vi "Euclidean_distances.vi"(6 "Type Y":T1(ring), 7 "Type X":T1(ring), 8 "error in":errorcluster caption="entrée d'erreur", 9 "Y":string[][](array[string]), 10 "X":string[][](array[string]), 11 "euclidean_distances":T3) -> (0 "error out":errorcluster caption="sortie d'erreur", 3 "Data":T2)   [LabVIEW 2020]
doc: "Considering the rows of X (and Y=X) as vectors, compute the distance matrix between each pair of vectors.\n\nFor efficiency reasons, the euclidean distance between a pair of row vector x and y is computed as :\n\ndist(x, y) = sqrt(dot(x, x) - 2 * dot(x, y) + dot(y, y))\n\nThis formulation has two advantages over other ways of computing distances. First, it is computationally efficient when dealing with sparse data. Second, if one argument varies but the other remains unchanged, then dot(x, x) and/or dot(y, y) can be pre-computed.\n\nHowever, this is not the most precise way of doing this computation, and the distance matrix returned by this function may not be exactly symmetric as required by, e.g., scipy.spatial.distance functions.\n\n\nParameters :\n\n- X : {array-like, sparse matrix}, shape (n_samples_1, n_features)\n\n- Y : {array-like, sparse matrix}, shape (n_samples_2, n_features)\n\n- Y_norm_squared : array-like, shape (n_samples_2, ), optional\nPre-computed dot-products of vectors in Y (e.g., (Y**2).sum(axis=1)) May be ignored in some cases, see the note below.\n\n- squared : boolean, optional\nReturn squared Euclidean distances.\n\n- X_norm_squared : array-like of shape (n_samples,), optional\nPre-computed dot-products of vectors in X (e.g., (X**2).sum(axis=1)) May be ignored in some cases, see the note below.\n\nReturns : \n\n- distances : array, shape (n_samples_1, n_samples_2)"
uses:
  Euclidean_distances.lvclass
panel:
  out "Euclidean_distances.lvclass":refnum<class "Euclidean_distances.lvclass">
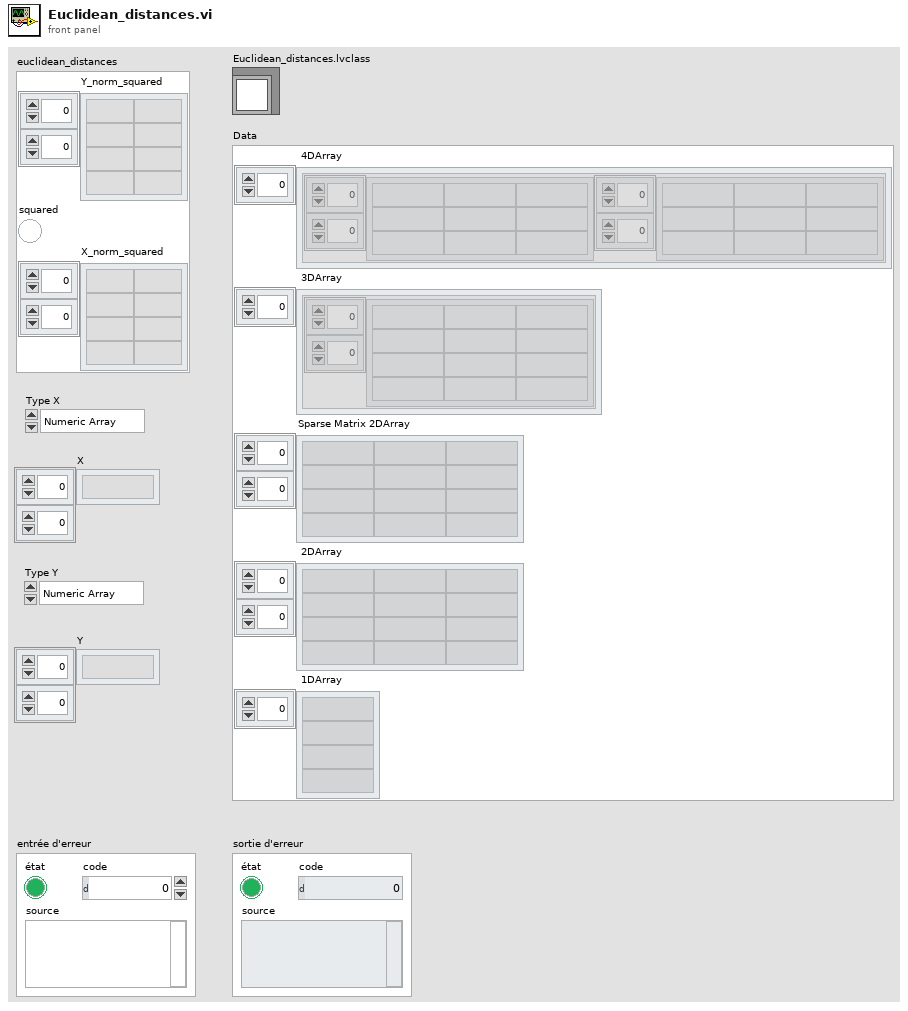
[diagram p1: front panel]
types:
  T1 = enum16{"Numeric Array", "String Array", "Sparse"}
  T2 = cluster{" 4DArray":cluster{"1":string[][], "2":string[][]}[], " 3DArray":cluster{"Tableau":string[][]}[], "Sparse Matrix 2DArray":string[][], " 2DArray":string[][], " 1DArray":string[]}
  T3 = cluster{"Y_norm_squared":string[][], "squared":bool, "X_norm_squared":string[][]}
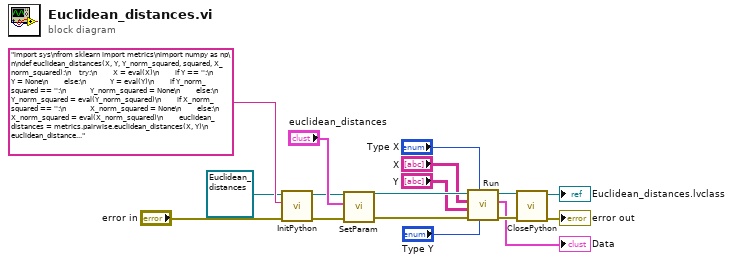
[diagram p0: block diagram]
diagram:
  n1 = call-dynamic "InitPython.vi"("error in (no error)"="error in", "Python Instruction"="import sys\nfrom sklearn import metrics\nimport numpy as np\n\ndef euclidean_distances(X, Y, Y_norm_squared, squared, X_norm_squared):\n    try:\n        X = eval(X)\n        if Y == '':\n            Y = None\n        else:\n            Y = eval(Y)\n        if Y_norm_squared == '':\n            Y_norm_squared = None\n        else:\n            Y_norm_squared = eval(Y_norm_squared)\n        if X_norm_squared == '':\n            X_norm_squared = None\n        else:\n            X_norm_squared = eval(X_norm_squared)\n        euclidean_distances = metrics.pairwise.euclidean_distances(X, Y)\n        euclidean_distances = euclidean_distances.tolist()\n        return str(euclidean_distances)\n    except:\n        erreur = sys.exc_info()\n        typerr = u\"%s\" % (erreur[0])\n        typerr = typerr[typerr.find(\"'\")+1:typerr.rfind(\"'\")]\n        msgerr = u\"%s\" % (erreur[1])\n        message = str('/!\\\\ {0} : {1}'. format(typerr,msgerr))\n        return message", "Scikit-learn en entrée"=refnum<class "Euclidean_distances.lvclass"> refnum ("Euclidean_distances.lvclass")) -> ("error out"=w13:errorcluster, "Scikit-learn en sortie"=w12:refnum<class "Euclidean_distances.lvclass">)  [unwired: 7 in]
  n2 = call-dynamic "SetParam.vi"("error in (no error)"=w13, "euclidean_distances"="euclidean_distances", "Euclidean_distances.lvclass"=w12) -> ("error out"=w8:errorcluster, "Euclidean_distances.lvclass"=w9:refnum<class "Euclidean_distances.lvclass">)  [unwired: 7 in]
  n3 = call-dynamic "Run.vi"("Type Y"="Type Y", "Type X"="Type X", "error in (no error)"=w8, "Y"="Y", "X"="X", "Euclidean_distances.lvclass"=w9) -> ("error out"=w10:errorcluster, "Data"=→"Data":T2, "Euclidean_distances.lvclass"=w11:refnum<class "Euclidean_distances.lvclass">)  [unwired: 3 in]
  n4 = call-dynamic "ClosePython.vi"("error in (no error)"=w10, "Scikit-learn en entrée"=w11) -> ("error out"=→"error out":errorcluster, "Scikit-learn en sortie"=→"Euclidean_distances.lvclass":refnum<class "Euclidean_distances.lvclass">)  [unwired: 8 in]
